vi "niFpgaPID_PIDWrapper.vi"(0 "setpoint":sgl, 1 "reset? (F)":bool, 3 "channel (0)":u8, 5 "process variable":sgl, 7 "manual control":T5, 12 "gains":T4 {"filter coefficient" min=0 max=1; "proportional gain" step=0.125}, 13 "output range":T3={"output high (Inf)"=inf, "output low (-Inf)"=-inf}, 14 "setpoint weighting":T2={"proportional weighting (1)"=1.0, "derivative weighting (0)"=0.0} {"derivative weighting (0)" min=0 max=1; "proportional weighting (1)" min=0 max=1}) -> (4 "output":sgl, 6 "error":sgl, 8 "actions":T1)   [LabVIEW 2017]
doc: "Implements a single-precision floating-point PID algorithm for PID applications with high-speed control and/or high channel count on an FPGA target. You can use this VI to create single-channel, multi-channel, and multi-rate control applications."
uses:
  <vilib>/rvi/Analysis/control/PID/Typedef/niFpgaPID_ManualControl.ctl
  <vilib>/rvi/Analysis/control/PID/Typedef/niFpgaPID_PIDGains.ctl
  <vilib>/rvi/Analysis/control/PID/Typedef/niFpgaPID_OutputRange.ctl
  <vilib>/rvi/Analysis/control/PID/Typedef/niFpgaPID_SetpointWeightings.ctl
  <vilib>/rvi/Analysis/control/PID/Typedef/niFpgaPID_PIDActions.ctl
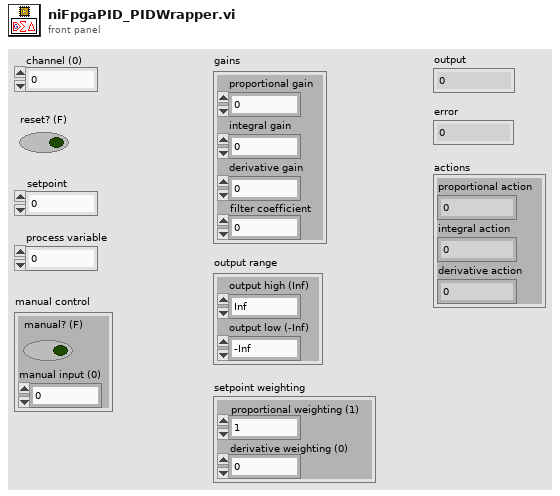
[diagram p1: front panel]
types:
  T1 = typedef "niFpgaPID_PIDActions.ctl" = cluster{"proportional action":sgl, "integral action":sgl, "derivative action":sgl}
  T2 = typedef "niFpgaPID_SetpointWeightings.ctl" = cluster{"proportional weighting (1)":sgl, "derivative weighting (0)":sgl}
  T3 = typedef "niFpgaPID_OutputRange.ctl" = cluster{"output high (Inf)":sgl, "output low (-Inf)":sgl}
  T4 = typedef "niFpgaPID_PIDGains.ctl" = cluster{"proportional gain":sgl, "integral gain":sgl, "derivative gain":sgl, "filter coefficient":sgl}
  T5 = typedef "niFpgaPID_ManualControl.ctl" = cluster{"manual? (F)":bool, "manual input (0)":sgl}
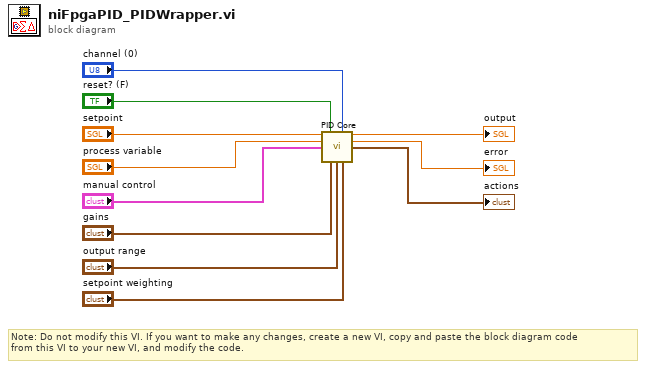
[diagram p0: block diagram]
diagram:
  # "Note: Do not modify this VI. If you want to make any changes, create a new VI, copy and paste the block diagram code\nfrom this VI to your new VI, and modify the code."
  n1 = call "PID Core"("setpoint"="setpoint", "reset? (F)"="reset? (F)", "channel (0)"="channel (0)", "process variable"="process variable", "manual control"="manual control", "gains"="gains", "output range"="output range", "setpoint weighting"="setpoint weighting") -> ("output"=→"output":sgl, "error"=→"error":sgl, "actions"=→"actions":T1)  [unwired: 5 in]
